vi "Decorator.vi"(8 "error in (no error)":errorcluster, 11 "Child in":refnum<class "Child.lvclass">) -> (0 "error out":errorcluster, 3 "Child out":refnum<class "Child.lvclass">)   [LabVIEW 2021, in "Child.lvclass"]
uses:
  Child.lvclass
  Parent/Parent.lvclass
  C:/PPLs/Composition-Approach/Template Method with Interfaces/Interface/Interface.lvclass
  Child.lvclass/Child.ctl
  C:/PPLs/Composition-Approach/Template Method with Interfaces/Interface 1/Interface 1.lvclass
  C:/PPLs/Composition-Approach/Template Method with Interfaces/Interface 2/Interface 2.lvclass
  C:/PPLs/Composition-Approach/Template Method with Interfaces/Parent/Parent.lvclass
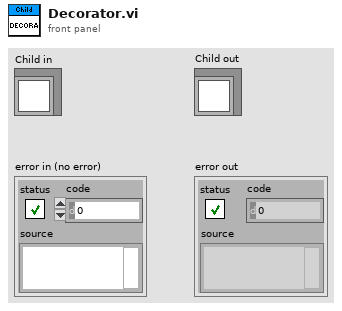
[diagram p1: front panel]
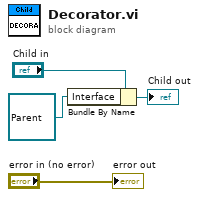
[diagram p0: block diagram]
diagram:
  n1 = Bundle By Name(cluster="Child in", "Interface"=refnum<class "Parent.lvclass"> refnum ("Parent.lvclass")) -> (→"Child out":refnum<class "Child.lvclass">)
  "error out" <- "error in (no error)"
